vi "Decode.vi"(8 "error in":errorcluster, 9 "input string":string, 11 "previous_Data":refnum<class "Data.lvclass">) -> (0 "error out":errorcluster, 3 "Data":refnum<class "Data.lvclass">)   [LabVIEW 2020, in "Data.lvclass"]
uses:
  Data.lvclass
  Data.lvclass/Data.ctl
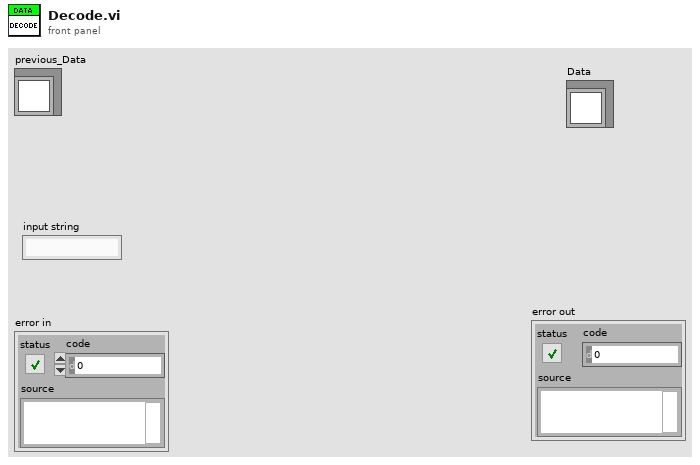
[diagram p1: front panel]
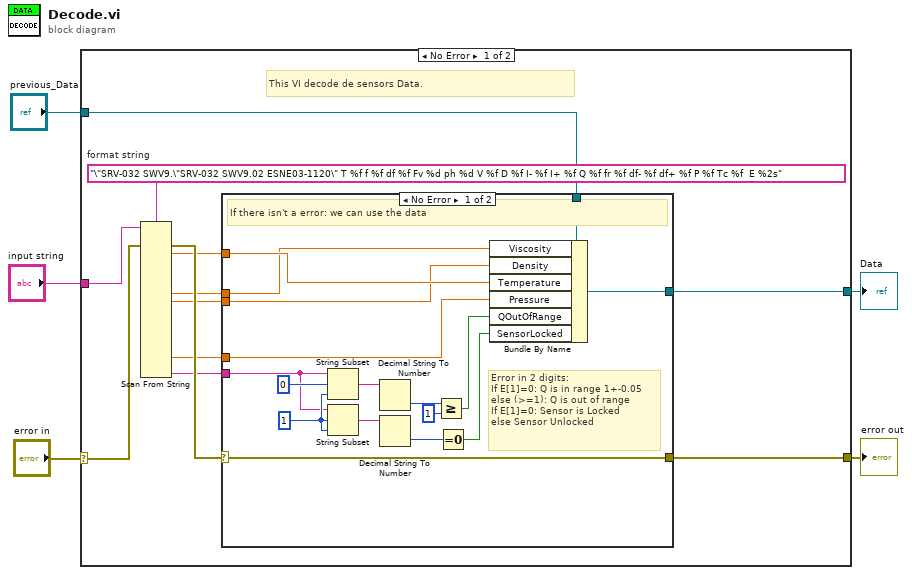
[diagram p0: block diagram]
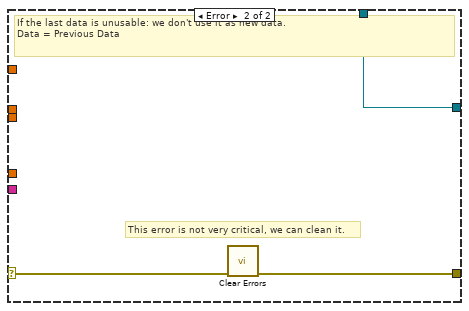
[diagram p2: hidden frame]
diagram:
  n1 = case shown="No Error" "error in" {
    selector: "error in" -> [w7 w39]
    tunnel: "input string" -> [w17 _]
    tunnel: "previous_Data" -> [w15 w38]
    tunnel: [w8 w38] -> w3
    tunnel: [w6 w39] -> w1
    frame No Error {
      w16 = "\"SRV-032 SWV9.\"SRV-032 SWV9.02 ESNE03-1120\" T %f f %f df %f Fv %d ph %d V %f D %f I- %f I+ %f Q %f fr %f df- %f df+ %f P %f Tc %f  E %2s"  # format string
      # "This VI decode de sensors Data."
      n2 = Scan From String(format string=w16, input string=w17, error in=w7) -> (error out=w14:errorcluster, output 1=w12:dbl, output 6=w13:dbl, output 7=w11:dbl, output 14=w9:dbl, output 16=w10:string)  [unwired: 28 in, 2 out]
      n3 = case shown="No Error" w14 {
        selector: w14 -> [w18 w36]
        tunnel: w15 -> [w34 w37]
        tunnel: w13 -> [w20 _]
        tunnel: w12 -> [w33 _]
        tunnel: w11 -> [w32 _]
        tunnel: w10 -> [w29 _]
        tunnel: w9 -> [w19 _]
        tunnel: [w21 w37] -> w8
        tunnel: [w18 w35] -> w6
        frame No Error {
          w30 = 1 ("length (rest)")
          # "Error in 2 digits:\nIf E[1]=0: Q is in range 1+-0.05\nelse (>=1): Q is out of range\nIf E[1]=0: Sensor is Locked\nelse Sensor Unlocked"
          # "If there isn't a error: we can use the data"
          n4 = String Subset(string=w29, offset (0)=0, length (rest)=w30) -> (substring=w28:string)
          n5 = String Subset(string=w29, offset (0)=w30, length (rest)=w30) -> (substring=w27:string)
          n6 = Decimal String To Number(string=w28) -> (number=w26:i32)  [unwired: 2 in, 1 out]
          n7 = Decimal String To Number(string=w27) -> (number=w23:i32)  [unwired: 2 in, 1 out]
          n8 = Greater Or Equal?(x=w26, y=1) -> (x >= y?=w24:bool)
          n9 = Equal To 0?(x=w23) -> (x = 0?=w22:bool)
          n10 = Bundle By Name(cluster=w34, "Viscosity"=w20, "Density"=w32, "Temperature"=w33, "Pressure"=w19, "QOutOfRange"=w24, "SensorLocked"=w22) -> (w21:refnum<class "Data.lvclass">)
        }
        frame Error {
          # "This error is not very critical, we can clean it."
          # "If the last data is unusable: we don't use it as new data.\nData = Previous Data"
          n11 = call <vilib>:"Clear Errors.vi"("error in (no error)"=w36) -> ("error out"=w35:errorcluster)  [unwired: 5 in, 1 out]
        }
      }
    }
    frame Error {
    }
  }
  "Data" <- w3
  "error out" <- w1
